vi "Main VI Stand-Alone Prevent Trip.vi"() -> ()   [LabVIEW 2020]
panel:
  out "channel 4 currents":dbl[](array[numeric])
  out "channel 3 currents":dbl[](array[numeric])
  out "channel 2 currents":dbl[](array[numeric])
  out "channel 1 currents":dbl[](array[numeric])
  in  "stop":bool
  out "Power Supply Trip":bool
  in  "Power Supply \nAddress":refnum<visa-resource-name>
  in  "Barcodes in":string[](array[string])
  in  "Barcodes in 2":string[](array[string])
  in  "Barcodes in 3":string[](array[string])
  in  "Barcodes in 4":string[](array[string])
  out "Elapsed Time (s)":dbl
  in  "Start":bool
  out "Test Is Running (Red)\nTest Is Stopped (Green)":bool
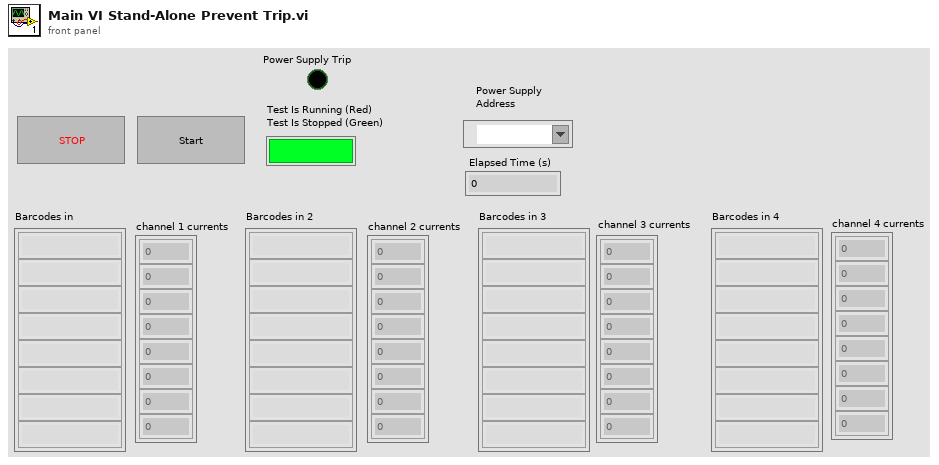
[diagram p1: front panel]
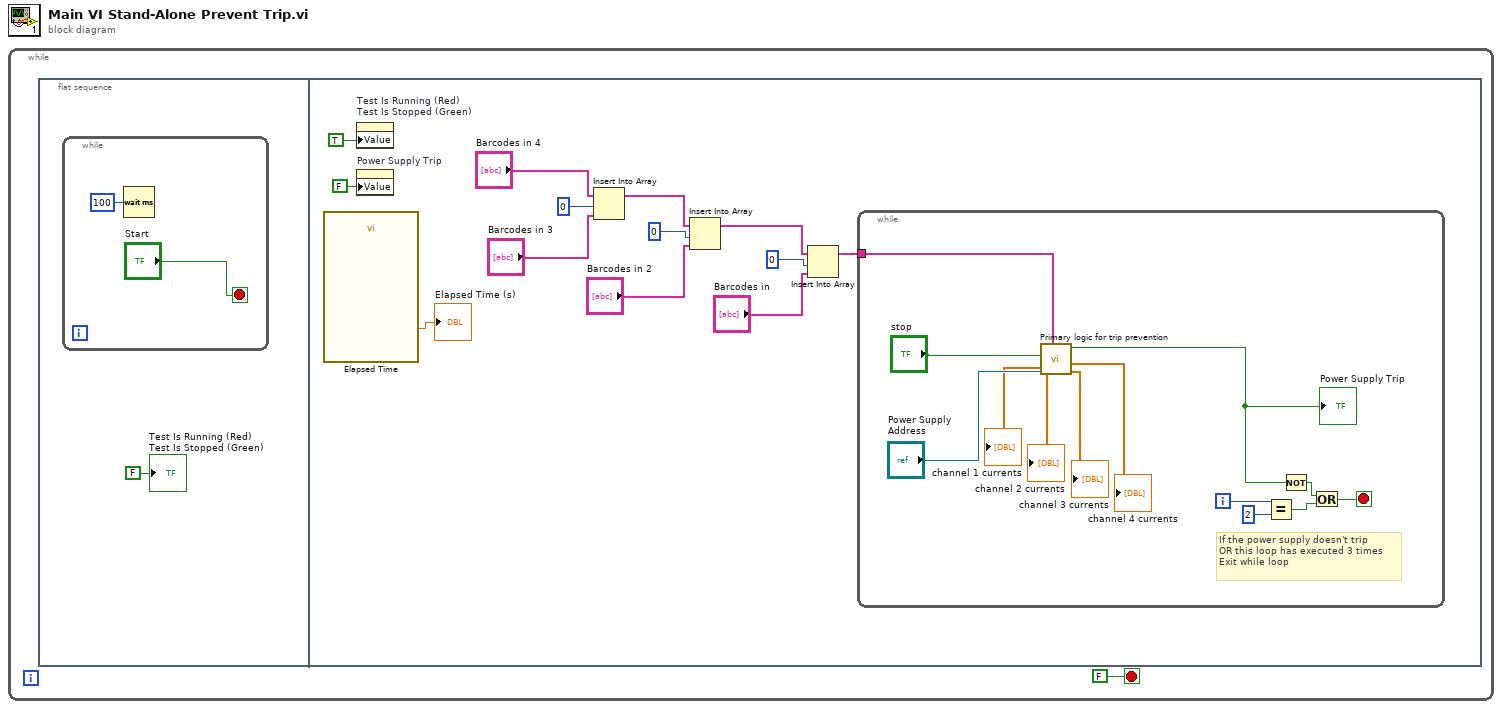
[diagram p0: block diagram]
diagram:
  n1 = while {
    stop <- FALSE stop-if-true
    n2 = flat-sequence {
      frame #0 {
        n3 = while {
          stop <- "Start" stop-if-true
          n4 = Wait (ms)(milliseconds to wait=u32 100) -> ()  [unwired: 1 out]
        }
        "Test Is Running (Red)\nTest Is Stopped (Green)" <- FALSE ("Start LED")
      }
      frame #1 {
        n5 = call "Elapsed Time"() -> ("Elapsed Time (s)"=→"Elapsed Time (s)":dbl)  [unwired: 12 in, 7 out]
        n6 = property on="Test Is Running (Red)\nTest Is Stopped (Green)" class="Bool (strict)"("Value"=TRUE) -> ()  [unwired: 2 in, 2 out]
        n7 = property on="Power Supply Trip" class="Bool (strict)"("Value"=FALSE ("Power Supply Trip")) -> ()  [unwired: 2 in, 2 out]
        n8 = Insert Into Array(array="Barcodes in 4", index=0, new element="Barcodes in 3") -> (w11:string[])
        n9 = Insert Into Array(array=w11, index=0, new element="Barcodes in 2") -> (w7:string[])
        n10 = Insert Into Array(array=w7, index=0, new element="Barcodes in") -> (w6:string[])
        n11 = while {
          tunnel: w6 -> [w22]
          i -> [w29]
          stop <- w26 stop-if-true
          # "If the power supply doesn't trip\nOR this loop has executed 3 times Exit while loop"
          n12 = call "Primary logic for trip prevention.vi"("Barcodes in"=w22, "VISA Refnum in"="Power Supply \nAddress", "Stop Program"="stop") -> ("channel 3 currents"=→"channel 3 currents":dbl[], "channel 4 currents"=→"channel 4 currents":dbl[], "Power Supply Trip"=w23:bool, "channel 2 currents"=→"channel 2 currents":dbl[], "channel 1 currents"=→"channel 1 currents":dbl[])  [unwired: 4 in]
          "Power Supply Trip" <- w23
          n13 = Equal?(x=w29, y=2) -> (x = y?=w27:bool)
          n14 = Not(x=w23) -> (.not. x?=w30:bool)
          n15 = Or(x=w30, y=w27) -> (x .or. y?=w26:bool)
        }
      }
    }
  }
